vi "Lookup Comment.vi"(3 "String in":string) -> (0 "Value":string, 1 "Comment":string)   [LabVIEW 2021, in "UDP_Config.lvclass"]
uses:
  UDP_Config.lvclass
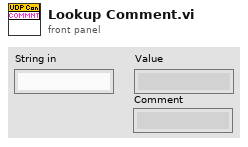
[diagram p1: front panel]
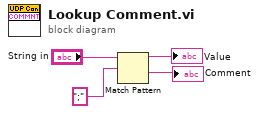
[diagram p0: block diagram]
diagram:
  n1 = Match Pattern(string="String in", regular expression=";" ("search string/char (-)")) -> (before substring=→"Value":string, after substring=→"Comment":string)  [unwired: 1 in, 2 out]
